vi "Read Origin Left.vi"(8 "error in (no error)":errorcluster, 11 "Picture.lvclass in":refnum<class "Picture.lvclass">) -> (0 "error out":errorcluster, 2 "Left":i16, 3 "Picture.lvclass out":refnum<class "Picture.lvclass">)   [LabVIEW 2015, in "Picture.lvclass"]
uses:
  Picture.lvclass
  Picture.lvclass/Picture.ctl
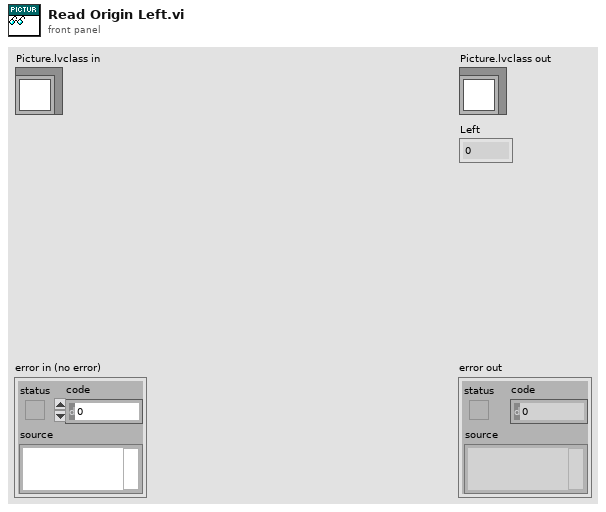
[diagram p1: front panel]
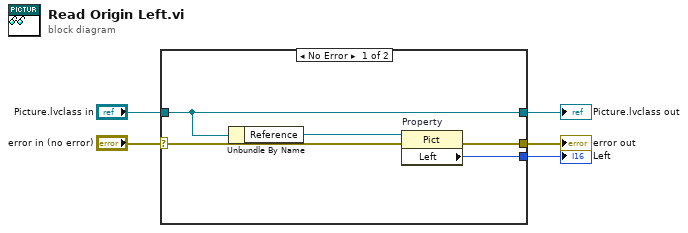
[diagram p0: block diagram]
diagram:
  n1 = case shown="No Error" "error in (no error)" {
    selector: "error in (no error)" -> [w6 w12]
    tunnel: [w9 w12] -> w4
    tunnel: [w8 w11] -> w2
    tunnel: "Picture.lvclass in" -> [w8 w11]
    tunnel: [w10 _] -> w1
    frame No Error {
      n2 = Unbundle By Name(w8) -> ("Reference"=w7:refnum<vi>)
      n3 = property on="Property" class="Pict"(reference=w7, error in=w6) -> (error out=w9:errorcluster, "Left"=w10:i16)  [unwired: 1 out]
    }
    frame Error {
    }
  }
  "error out" <- w4
  "Picture.lvclass out" <- w2
  "Left" <- w1
